vi "Create.vi"(7 "VolatusAPI":refnum<class "VolatusAPI.lvclass">, 8 "error in (no error)":errorcluster, 10 "Inhibit Channel":string, 11 "Control Ref":refnum<vi>) -> (0 "error out":errorcluster, 3 "Element Inhibit out":refnum<class "Element Inhibit.lvclass">)   [LabVIEW 2020, in "VolatusGUI.lvlib" / "Element Inhibit.lvclass"]
uses:
  Element Inhibit.lvclass
  Element Inhibit.lvclass/Element Inhibit.ctl
  Volatus/VolatusAPI/VolatusAPI.lvclass
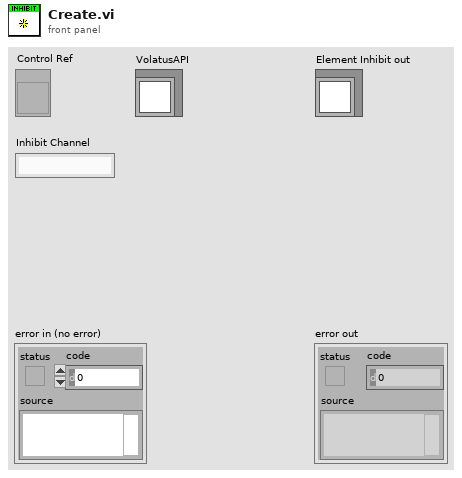
[diagram p1: front panel]
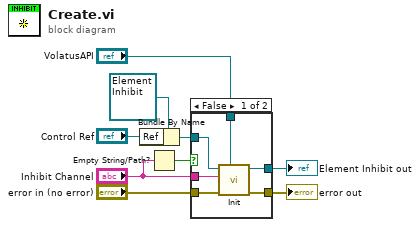
[diagram p0: block diagram]
diagram:
  n1 = Bundle By Name(cluster=refnum<class "Element Inhibit.lvclass"> refnum ("Element Inhibit in"), "Ref"="Control Ref") -> (w5:refnum<class "Element Inhibit.lvclass">)
  n2 = Empty String/Path?(string/path="Inhibit Channel") -> (empty?=w3:bool)
  n3 = case shown="False" w3 {
    tunnel: "error in (no error)" -> [w15 w16]
    tunnel: [w14 w16] -> w6
    tunnel: w5 -> [w13 w17]
    tunnel: [w12 w17] -> w4
    tunnel: "VolatusAPI" -> [w11 _]
    tunnel: "Inhibit Channel" -> [w10 _]
    frame False {
      n4 = call "Init.vi"("VolatusAPI"=w11, "error in (no error)"=w15, "Inhibit Channel"=w10, "Element Inhibit in"=w13) -> ("error out"=w14:errorcluster, "Element Inhibit out"=w12:refnum<class "Element Inhibit.lvclass">)  [unwired: 6 in]
    }
    frame True {
    }
  }
  "error out" <- w6
  "Element Inhibit out" <- w4
